vi "Alias to Q.vi"(10 "Msg Q DVR Alias":string, 11 "Self Actor in":refnum<class "Self Actor.lvclass">) -> (0 "error out":errorcluster, 2 "Nested Msg Q DVR":refnum<data-value>)   [LabVIEW 2021, in "jettl.lvlib" / "Self Actor.lvclass"]
uses:
  Self Actor.lvclass
  Msg Strategy/Msg Strategy.lvclass
  Self Actor.lvclass/Self Actor.ctl
  jettl.lvlib
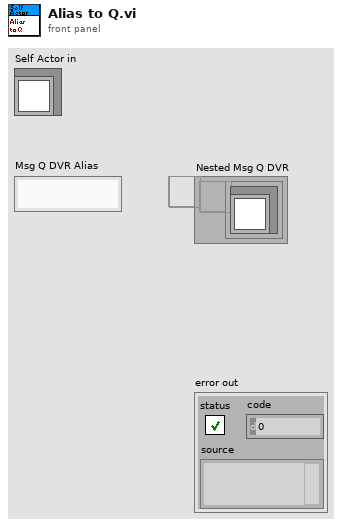
[diagram p1: front panel]
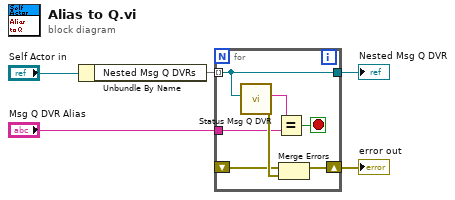
[diagram p0: block diagram]
diagram:
  n1 = Unbundle By Name("Self Actor in") -> ("Nested Msg Q DVRs"=w4:set{refnum<data-value>})
  n2 = for {
    tunnel: w4 -> [w12] mode=indexing
    tunnel: [w12] -> w2
    tunnel: "Msg Q DVR Alias" -> [w6]
    shift-right: [w7] -> w1
    shift-left: _ -> [w8]
    stop <- w9 stop-if-true
    n3 = call "Status Msg Q DVR.vi"("Msg Q DVR"=w12) -> ("error out"=w10:errorcluster, "Msg Q DVR Alias"=w11:string)  [unwired: 9 in]
    n4 = Equal?(x=w11, y=w6) -> (x = y?=w9:bool)
    n5 = Merge Errors(w8, w10) -> (w7:errorcluster)
  }
  "error out" <- w1
  "Nested Msg Q DVR" <- w2
